vi "MFLI set default parameters.vi"(8 "error in (no error)":errorcluster, 11 "Lock-in Handle":T1 {"Handle" format="0x%08x"; "Conn" format="0x%08x"}) -> (0 "Error Out":errorcluster, 3 "Handle Out":T1 {"Handle" format="0x%08x"; "Conn" format="0x%08x"})   [LabVIEW 2022 SP3, in "Lock-in module.lvlib"]
uses:
  Lock-in module.lvlib
  <instrlib>/Zurich Instruments LabOne/Public/ziTypeHandle.ctl
  <instrlib>/Zurich Instruments LabOne/Public/Configure/ziSetValueDoubleArray.vi
  <instrlib>/Zurich Instruments LabOne/Zurich Instruments LabOne.lvlib
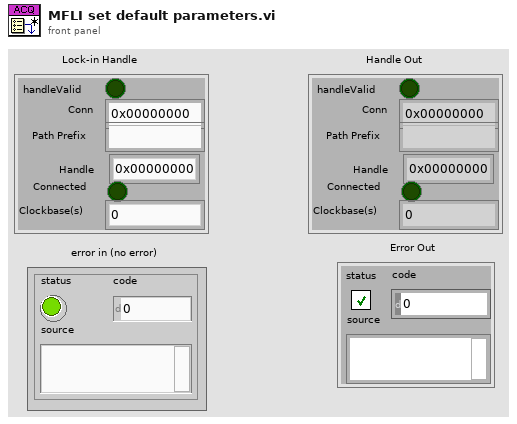
[diagram p1: front panel]
types:
  T1 = typedef "Zurich Instruments LabOne.lvlib/ziTypeHandle.ctl" = cluster{"handleValid":bool, "Conn":u64, "Path Prefix":string, "Handle":u64, "Connected":bool, "Clockbase(s)":dbl}
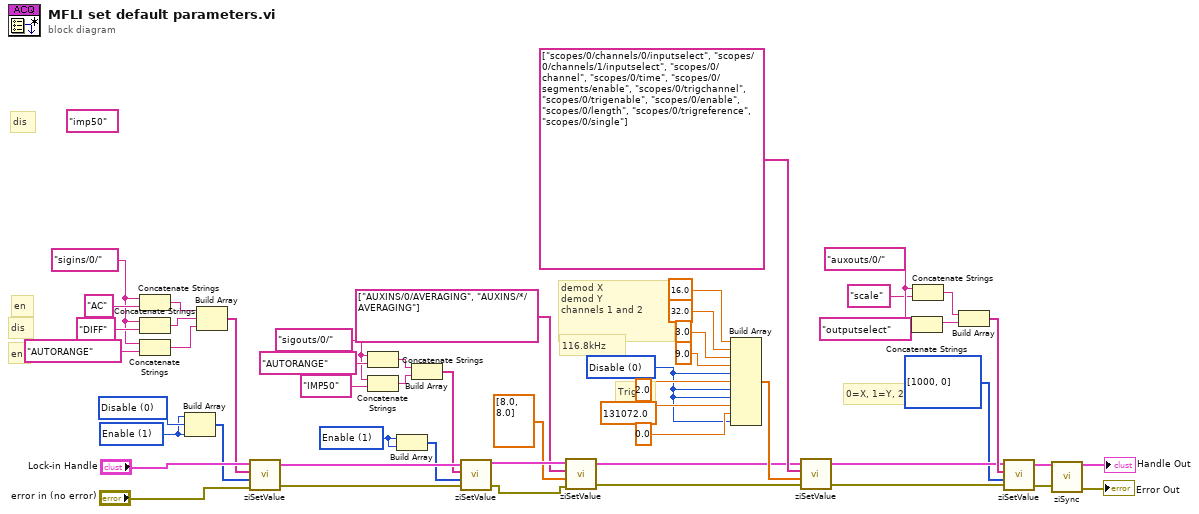
[diagram p0: block diagram]
diagram:
  w23 = "auxouts/0/" ("string")
  w7 = u16 0 items=["Disable", "Enable"]
  w27 = u16 1 items=["Disable", "Enable"]
  w36 = u16 0 items=["Disable", "Enable"]
  w33 = u16 1 items=["Disable", "Enable"]
  w47 = "sigouts/0/" ("string")
  (unwired) "imp50" ("Path")
  w50 = "sigins/0/"
  # "en"
  # "dis"
  # "en"
  # "dis"
  # "Trig1"
  # "116.8kHz"
  # "demod X\ndemod Y\nchannels 1 and 2"
  # "0=X, 1=Y, 2=R"
  n1 = Concatenate Strings(w50, "AC" ("Path")) -> (w39:string)
  n2 = Concatenate Strings(w50, "DIFF" ("Path")) -> (w38:string)
  n3 = Concatenate Strings(w50, "AUTORANGE" ("Path")) -> (w37:string)
  n4 = Build Array(w33, w36, w33) -> (w34:u16[])
  n5 = Build Array(w39, w38, w37) -> (w35:string[])
  n6 = call-poly <instrlib>:"ziSetValue.vi"("Error In"="error in (no error)", "Values"=w34, "Paths"=w35, "Handle In"="Lock-in Handle") -> ("Error Out"=w31:errorcluster, "Handle Out"=w32:T1)  [unwired: 1 in]
  n7 = Concatenate Strings(w47, "AUTORANGE" ("Path")) -> (w30:string)
  n8 = Concatenate Strings(w47, "IMP50" ("Path")) -> (w29:string)
  n9 = Build Array(w27, w27) -> (w26:u16[])
  n10 = Build Array(w30, w29) -> (w28:string[])
  n11 = call-poly <instrlib>:"ziSetValue.vi"("Error In"=w31, "Values"=w26, "Paths"=w28, "Handle In"=w32) -> ("Error Out"=w6:errorcluster, "Handle Out"=w4:T1)  [unwired: 1 in]
  n12 = call-poly <instrlib>:"ziSetValue.vi"("Error In"=w6, "Values"=dbl[] [8.0, 8.0], "Paths"=string[] ["AUXINS/0/AVERAGING", "AUXINS/*/AVERAGING"] ("Path"), "Handle In"=w4) -> ("Error Out"=w5:errorcluster, "Handle Out"=w3:T1)  [unwired: 1 in]
  n13 = Build Array(16.0 ("element"), 32.0 ("element"), 3.0 ("element"), 9.0 ("element"), w7, 2.0 ("element"), w7, w7, 131072.0 ("element"), 0.0 ("element"), w7) -> (w40:dbl[])
  n14 = call-poly <instrlib>:"ziSetValue.vi"("Error In"=w5, "Values"=w40, "Paths"=string[] ["scopes/0/channels/0/inputselect", "scopes/0/channels/1/inputselect", "scopes/0/channel", "scopes/0/time", "scopes/0/segments/enable", "scopes/0/trigchannel", "scopes/0/trigenable", "scopes/0/enable", "scopes/0/length", "scopes/0/trigreference", "scopes/0/single"], "Handle In"=w3) -> ("Error Out"=w11:errorcluster, "Handle Out"=w17:T1)  [unwired: 1 in]
  n15 = Concatenate Strings(w23, "outputselect") -> (w20:string)
  n16 = Concatenate Strings(w23, "scale" ("string")) -> (w21:string)
  n17 = Build Array(w21, w20) -> (w18:string[])
  n18 = call-poly <instrlib>:"ziSetValue.vi"("Error In"=w11, "Values"=i32[] [1000, 0], "Paths"=w18, "Handle In"=w17) -> ("Error Out"=w15:errorcluster, "Handle Out"=w16:T1)  [unwired: 1 in]
  n19 = call <instrlib>:"ziSync.vi"("Handle In"=w16, "Error In"=w15) -> ("Handle Out"=→"Handle Out":T1, "Error Out"=→"Error Out":errorcluster)  [unwired: 12 in]
